vi "Unicode (UCS32) to UTF16 Encoding.vi"(8 "error in":errorcluster, 9 "[UCS 32]":u32=2949 format="%.0x") -> (0 "error out":errorcluster, 1 "[UTF-16]":u16[](array[numeric])=[2949] format="%.0x")   [LabVIEW 2011]
doc: "Encodes the given Unicode number in UTF16 format."
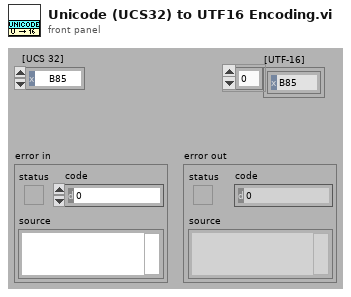
[diagram p1: front panel]
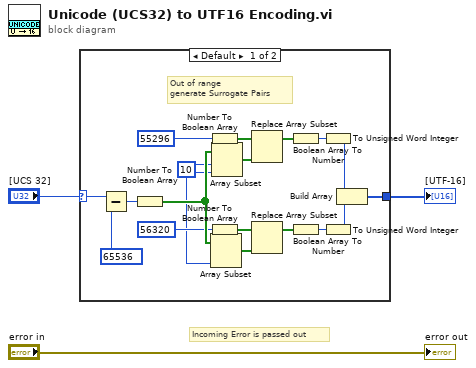
[diagram p0: block diagram]
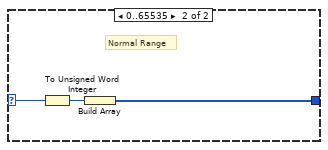
[diagram p2: hidden frame]
diagram:
  # "Incoming Error is passed out"
  n1 = case shown="Default" "[UCS 32]" {
    selector: "[UCS 32]" -> [w21 w24]
    tunnel: [w7 w22] -> w2
    frame Default {
      w6 = 10 ("length")
      # "Out of range \ngenerate Surrogate Pairs"
      n2 = Subtract(x=w21, y=u32 65536 ("unsigned 16bit integer")) -> (x-y=w19:u32)
      n3 = Number To Boolean Array(number=w19) -> (Boolean array=w18:bool[])
      n4 = Number To Boolean Array(number=u16 55296 ("unsigned 16bit integer")) -> (Boolean array=w16:bool[])
      n5 = Number To Boolean Array(number=u16 56320 ("unsigned 16bit integer")) -> (Boolean array=w14:bool[])
      n6 = Array Subset(array=w18, length=w6) -> (w4:bool[])  [unwired: 1 in]
      n7 = Array Subset(array=w18, index=w6, length=w6) -> (w5:bool[])
      n8 = Replace Array Subset(array=w16, new element=w5) -> (w12:bool[])  [unwired: 1 in]
      n9 = Replace Array Subset(array=w14, new element=w4) -> (w13:bool[])  [unwired: 1 in]
      n10 = Boolean Array To Number(Boolean array=w12) -> (number=w10:u32)
      n11 = Boolean Array To Number(Boolean array=w13) -> (number=w9:u32)
      n12 = To Unsigned Word Integer(number=w10) -> (unsigned 16bit integer=w11:u16)
      n13 = To Unsigned Word Integer(number=w9) -> (unsigned 16bit integer=w8:u16)
      n14 = Build Array(w11, w8) -> (w7:u16[])
    }
    frame 0..65535 {
      # "Normal Range"
      n15 = To Unsigned Word Integer(number=w24) -> (unsigned 16bit integer=w23:u16)
      n16 = Build Array(w23) -> (w22:u16[])
    }
  }
  "[UTF-16]" <- w2
  "error out" <- "error in"
